vi "Move.vi"(8 "error in (no error)":errorcluster, 11 "StageSPIM in":refnum<class "StageSPIM.lvclass">) -> (0 "error out":errorcluster, 3 "StageSPIM out":refnum<class "StageSPIM.lvclass">)   [LabVIEW 2012, in "StageSPIM.lvclass"]
uses:
  StageSPIM.lvclass
  StageSPIM.lvclass/StageSPIM.ctl
panel:
  out "Target position":dbl[][](array[numeric])
  out "Controller error":bool
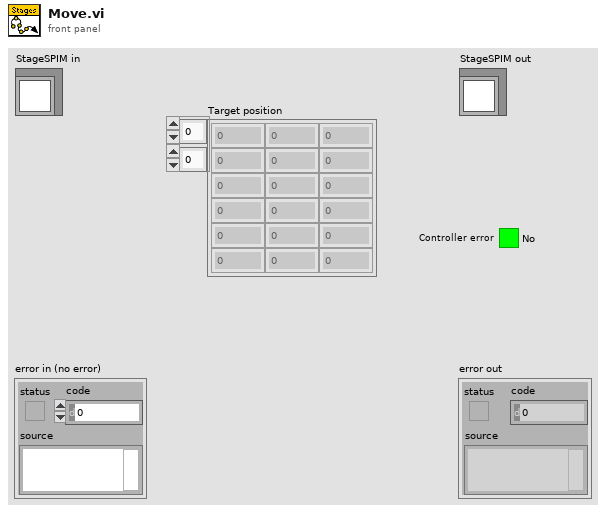
[diagram p1: front panel]
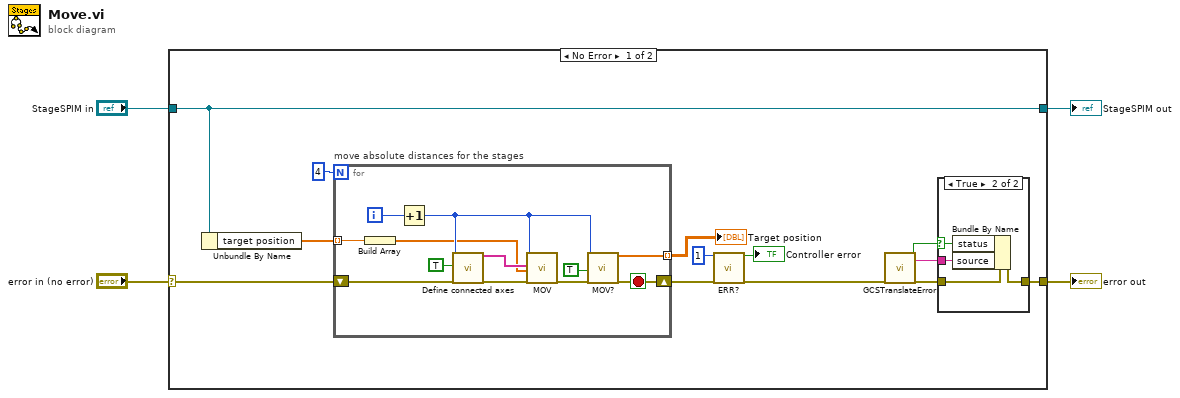
[diagram p0: block diagram]
diagram:
  n1 = case shown="No Error" "error in (no error)" {
    selector: "error in (no error)" -> [w16 w36]
    tunnel: [w8 w36] -> w3
    tunnel: [w15 w35] -> w1
    tunnel: "StageSPIM in" -> [w15 w35]
    frame No Error {
      n2 = Unbundle By Name(w15) -> ("target position"=w14:dbl[])
      n3 = for "move absolute distances for the stages" {
        N: 4 -> [_]
        shift-right: [w24] -> w13
        shift-left: w16 -> [w33]
        tunnel: w14 -> [w34] mode=indexing
        tunnel: [w23] -> w5 mode=indexing
        i -> [w32]
        stop <- w24 stop-if-true
        n4 = Build Array(w34) -> (w26:dbl[])
        n5 = Increment(x=w32) -> (x+1=w31:i32)
        n6 = call "Define connected axes.vi"("System no."=w31, "Read from\ncontroller?"=TRUE ("Read from\ncontroller?"), "error in"=w33) -> ("Conn. Axes out"=w27:string[], "error out"=w30:errorcluster)  [unwired: 15 in]
        n7 = call "MOV.vi"("System no."=w31, "Axes to move"=w27, "Position values"=w26, "error in"=w30) -> ("error out"=w29:errorcluster)  [unwired: 15 in]
        n8 = call "MOV?.vi"("System no."=w31, "All axes?"=TRUE, "error in"=w29) -> ("Target position"=w23:dbl[], "error out"=w24:errorcluster)  [unwired: 15 in]
      }
      "Target position" <- w5
      n9 = call "ERR?.vi"("System no."=1, "error in"=w13) -> ("Controller error"=→"Controller error":bool, "error out"=w12:errorcluster)  [unwired: 16 in]
      n10 = call "GCSTranslateError.vi"("error in"=w12) -> ("GCS Error?"=w7:bool, "Error Description"=w6:string, "error out"=w9:errorcluster)  [unwired: 16 in]
      n11 = case shown="True" w7 {
        selector: w7 -> [_ w20]
        tunnel: w9 -> [w18 w22]
        tunnel: [w18 w21] -> w8
        tunnel: w6 -> [_ w19]
        frame False {
        }
        frame True {
          n12 = Bundle By Name(cluster=w22, "status"=w20, "source"=w19) -> (w21:errorcluster)
        }
      }
    }
    frame Error {
    }
  }
  "error out" <- w3
  "StageSPIM out" <- w1
